vi "Snapshot.vi"() -> ()   [LabVIEW 2020]
uses:
  <vilib>/picture/picture.llb/Draw 8-Bit Pixmap.vi
  bin/gindustrialcam_64-1.so
panel:
  out "new picture":picture
  out "error out":errorcluster
  in  "error in (no error)":errorcluster
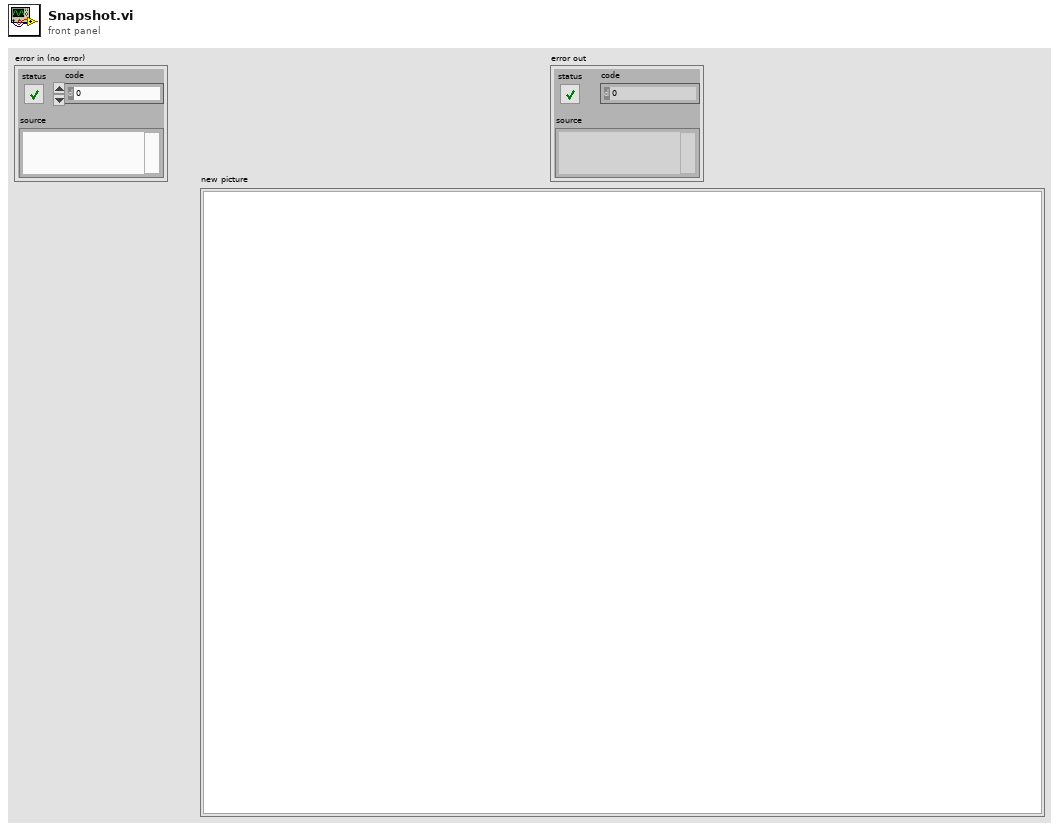
[diagram p1: front panel]
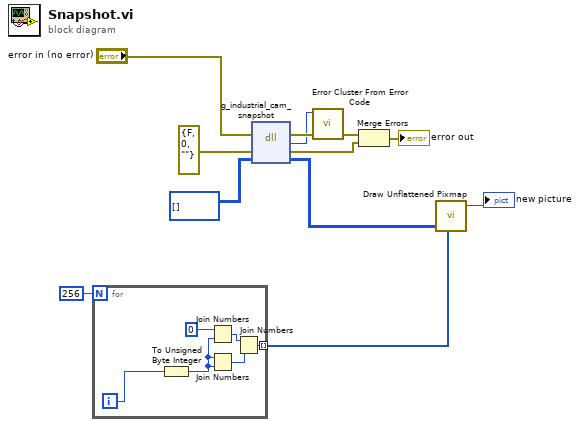
[diagram p0: block diagram]
diagram:
  n1 = for {
    N: 256 -> [_]
    tunnel: [w13] -> w2 mode=indexing
    i -> [w18]
    n2 = To Unsigned Byte Integer(number=w18) -> (unsigned 8bit integer=w17:u8)
    n3 = Join Numbers(hi=u8 0, lo=w17) -> ((hi.lo)=w15:u16)
    n4 = Join Numbers(hi=w17, lo=w17) -> ((hi.lo)=w14:u16)
    n5 = Join Numbers(hi=w15, lo=w14) -> ((hi.lo)=w13:u32)
  }
  n6 = dll-call lib="home/john/g-industrial-camera/LabVIEW/bin/gindustrialcam_*-1.*" fn="g_industrial_cam_snapshot"(error in="error in (no error)", "error"=errorcluster {"status"=FALSE, "code"=0, "source"=""} ("error constant"), "buffer"=u8[][] []) -> (error out=w11:errorcluster, "return type"=w10:i32, "error"=w6:errorcluster, "buffer"=w4:u8[][])  [unwired: 2 in, 1 out]
  n7 = call <vilib>:"Error Cluster From Error Code.vi"("error in (no error)"=w11, "error code (0)"=w10) -> ("error out"=w7:errorcluster)  [unwired: 7 in]
  n8 = Merge Errors(w7, w6) -> (→"error out":errorcluster)
  n9 = call-poly <vilib>:"Draw Unflattened Pixmap.vi"("data"=w4, "color table"=w2) -> ("new picture"=→"new picture":picture)  [unwired: 7 in]
